vi "mod_Double Changed (single).vi"(0 "input double":dbl format="%.2p") -> (1 "output double":dbl, 2 "changed?":bool)   [LabVIEW 2020, in "niAMT.lvlib"]
uses:
  <vilib>/addons/Modulation/niAMT.lvlib
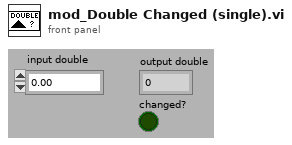
[diagram p1: front panel]
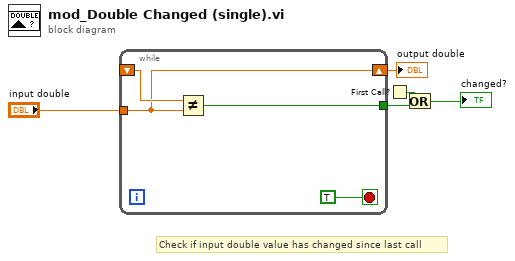
[diagram p0: block diagram]
diagram:
  # "Check if input double value has changed since last call"
  n1 = while {
    shift-right: [w7] -> w1
    shift-left: _ -> [w8]
    tunnel: "input double" -> [w7]
    tunnel: [w6] -> w3
    stop <- TRUE stop-if-true
    n2 = Not Equal?(x=w8, y=w7) -> (x != y?=w6:bool)
  }
  "output double" <- w1
  n3 = First Call?() -> (First Call?: T/F=w4:bool)
  n4 = Or(x=w4, y=w3) -> (x .or. y?=→"changed?":bool)
